vi "touch.vi"() -> ()   [LabVIEW 2015]
uses:
  <vilib>/NXT/Block Support/NXT_InputPort.ctl
  <vilib>/NXT/Dual Mode Library/Sensors/Touch_Pressed.vi
  <vilib>/NXT/Dual Mode Library/Motors/MotorReverse.vi
  <vilib>/NXT/Dual Mode Library/Waits/Wait_Num.vi
  <vilib>/NXT/Dual Mode Library/Motors/MotorOn.vi
panel:
  out "물체 감지":bool
  in  "stop":bool
  in  "Power (75)":i32=75
  in  "우 회전 시간":sgl=1.0
  in  "후진 시간":sgl=1.0
  in  "Port (Port 1)":T1 items=["Port 1", "Port 2", "Port 3", "Port 4"]
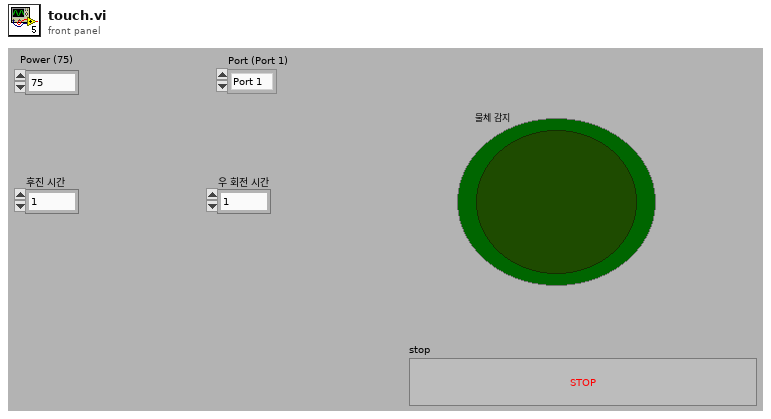
[diagram p1: front panel]
types:
  T1 = typedef "NXT_InputPort.ctl" = u32
  T2 = typedef "LVHSConnector.ctl" = refnum<class "BrickReference.lvclass">
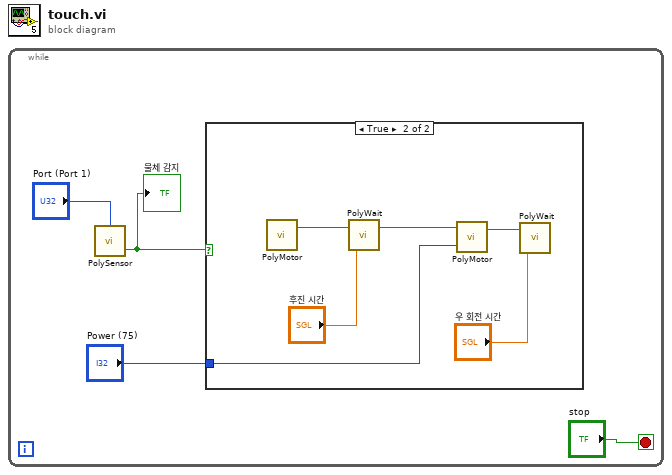
[diagram p0: block diagram]
diagram:
  n1 = while {
    stop <- "stop" stop-if-true
    n2 = call-poly <vilib>:"PolySensor.vi"("Port (Port 1)"="Port (Port 1)") -> ("Yes / No"=w1:bool)  [unwired: 2 in, 1 out]
    "물체 감지" <- w1
    n3 = case shown="True" w1 {
      tunnel: "Power (75)" -> [_ w5]
      frame False {
      }
      frame True {
        n4 = call-poly <vilib>:"PolyMotor.vi"() -> ("NXT/EV3"=w10:T2)  [unwired: 4 in]
        n5 = call-poly <vilib>:"PolyWait.vi"("Time (1 sec)"="후진 시간", "NXT/EV3"=w10) -> ("NXT/EV3"=w9:T2)  [unwired: 2 in]
        n6 = call-poly <vilib>:"PolyMotor.vi"("Power (75)"=w5, "NXT/EV3"=w9) -> ("NXT/EV3"=w8:T2)  [unwired: 2 in]
        n7 = call-poly <vilib>:"PolyWait.vi"("Time (1 sec)"="우 회전 시간", "NXT/EV3"=w8) -> ()  [unwired: 2 in, 1 out]
      }
    }
  }
